vi "MrClean.reset.vi"(0 "i ref in":refnum<vi>, 3 "ms timeout (100)":i32=100, 5 "error in (no error)":errorcluster) -> (14 "i ref out":refnum<vi>, 17 "timed out":bool, 19 "error out":errorcluster)   [LabVIEW 2014, in "MrClean.lvlib"]
doc: "Resets all function generators used by the CleanHandler. The function generators used by the CleanHandler are specified in the database"
uses:
  MrClean.lvlib
  CS_Core/CSSystem/CoreDefs/CoreDefs.error_type.ctl
  CS_Core/BaseProcess/BaseProcess.lvlib
  CS_Core/CSSystem/CoreLib/CoreLib.lvlib
  LEBITLib/LEBITLib.lvlib
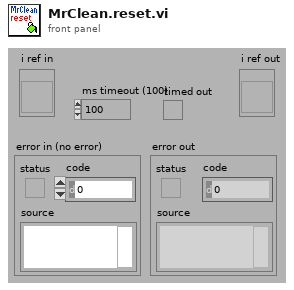
[diagram p1: front panel]
types:
  T1 = typedef "CoreDefs.error_type.ctl" = enum16{"no error", "can't load process", "can't unload process", "process does not exist", "can't install process", "can't remove process", "unknown function", "time out", "can't execute function", "duplicate queue name", "super not found", "caller queue invalid", "can't ping process", "unknown error", "VISA Error", "VISA timeout", "GPIB timeout", "GPIB error", "communication error", "data type mismatch", "can't read data from OPC server", "can't write data to OPC server", "OET error", "function not implemented", "process already exists", "invalid Shared Variable name", "error writing Shared Variable", "error reading Shared Variable", "invalid client name", "corrupt database", "unknown class", "call not authorized", "parameter out of range", "OET timeout: can't get data to modify", "invalid queue name", "requested operation incompatible with current state", "event undefined", "event disabled", "state undefined", "caller is not a friend", "EventBuilder: bad eventID", "EventBuilder: no DAQ devices", "a thread must not stop itself", "UNUSED ELEMENT4", "DiscArchiver: eventData incomplete", "DiscArchiver: eventData does not belong to run", "DiscArchiver: can't open file", "DiscArchiver: can't write to file", "DiscArchiver: available disc space low", "can't acquire semaphore", "error reading data from database", "notifier object is not existing", "can't register process", "can't unregister process", "illegal event type", "object disabled", "object already exists", "can't change state", "Instrument not found", "no connection to remote node", "invalid reference", "N/A", "UNUSED ELEMENT 1", "element not found", "illegal TCP/IP connection detected", "object does not exist", "invalid access ID", "unknown CS system", "invalid privilige", "unsupported data type", "unsupported server type", "IO server already exists", "Shared Variable already exists"}
  T2 = enum16{"simple", "synchronous", "asynchronous", "notification"}
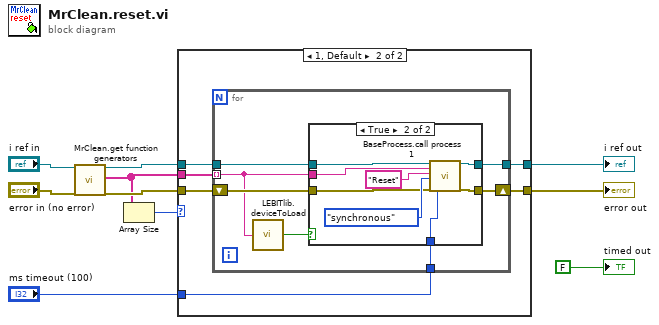
[diagram p0: block diagram]
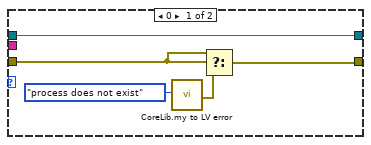
[diagram p2: hidden frame]
diagram:
  n1 = call "MrClean.get function generators.vi"("i ref in"="i ref in", "error in (no error)"="error in (no error)") -> ("i ref out"=w7:refnum<vi>, "function generators"=w3:string[], "error out"=w5:errorcluster)  [unwired: 14 in, 1 out]
  n2 = Array Size(array=w3) -> (size(s)=w8:i32)
  n3 = case shown="1, Default" w8 {
    tunnel: [w15 w19] -> w6
    tunnel: w7 -> [w15 w20]
    tunnel: [w13 w17] -> w4
    tunnel: w5 -> [w12 w18]
    tunnel: w3 -> [_ w21]
    tunnel: "ms timeout (100)" -> [_ w16]
    frame 0 {
      n4 = call "CoreLib.my to LV error.vi"("ErrorTypes"=CoreDefs.error_type."process does not exist") -> ("myErrorCluster"=w11:errorcluster)  [unwired: 17 in, 1 out]
      n5 = Select(t=w12, s=w12, f=w11) -> (s? t:f=w13:errorcluster)
    }
    frame 1, Default {
      n6 = for {
        tunnel: w21 -> [w22] mode=indexing
        tunnel: w20 -> [w28]
        tunnel: [w27] -> w19
        shift-right: [w25] -> w17
        shift-left: w18 -> [w26]
        tunnel: w16 -> [w24]
        n7 = call "LEBITlib.deviceToLoad.vi"("DeviceName"=w22) -> ("DeviceIsToLoad"=w23:bool)
        n8 = case shown="True" w23 {
          tunnel: w28 -> [w30 w38]
          tunnel: w22 -> [_ w36]
          tunnel: [w30 w34] -> w27
          tunnel: w26 -> [w29 w33]
          tunnel: [w29 w32] -> w25
          tunnel: w24 -> [_ w31]
          frame False {
          }
          frame True {
            n9 = call "BaseProcess.call process 1.vi"("i ref in"=w38, "Object"=w36, "Selector"="Reset", "CallType"=T2."synchronous", "error in (no error)"=w33, "timeout (ms)"=w31) -> ("i ref out"=w34:refnum<vi>, "error out"=w32:errorcluster)  [unwired: 11 in, 1 out]
          }
        }
      }
    }
  }
  "error out" <- w4
  "i ref out" <- w6
  "timed out" <- FALSE ("timed out")
